vi "信息转换.vi"(7 "联机模式":enum16{"单机", "追溯"}(ring)=enum."追溯", 8 "错误输入（无错误）":errorcluster, 10 "追溯码":string[](array[string]), 11 "测试信息":T1) -> (0 "错误输出":errorcluster, 3 "信息输出":string[](array[string]))   [LabVIEW 2020]
panel:
  # "用户信息转换"
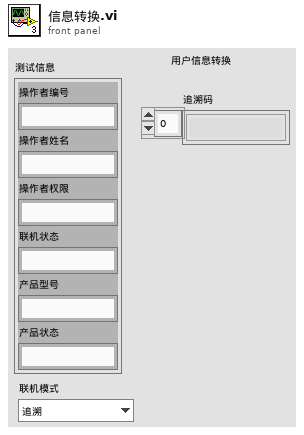
[diagram p1: front panel]
types:
  T1 = cluster{"操作者编号":string, "操作者姓名":string, "操作者权限":string, "联机状态":string, "产品型号":string, "产品状态":string}
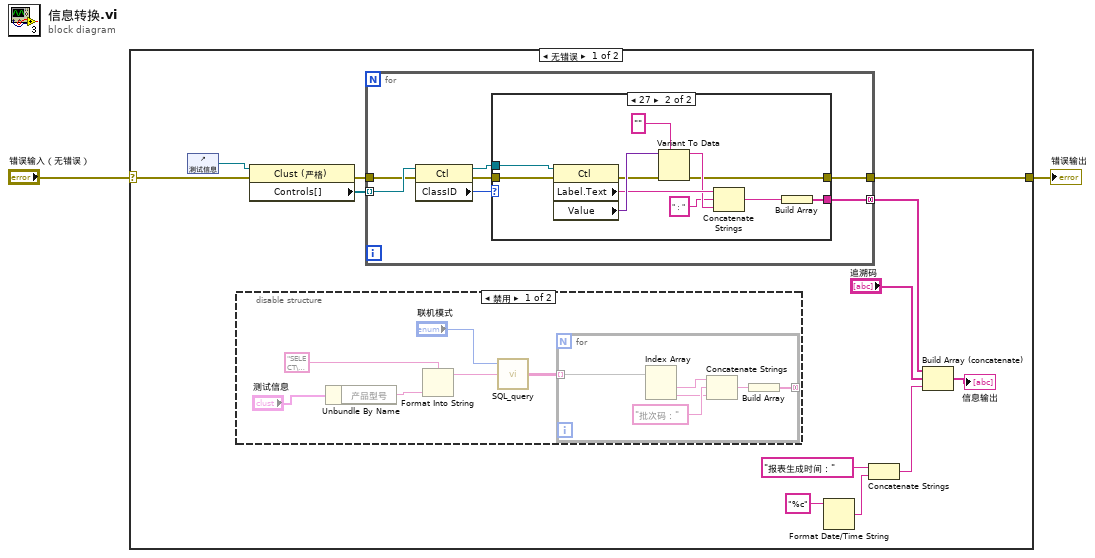
[diagram p0: block diagram]
diagram:
  n1 = case shown="无错误" "错误输入（无错误）" {
    selector: "错误输入（无错误）" -> [w7 w46]
    tunnel: [w5 w46] -> w1
    frame No Error {
      n2 = control-ref of="测试信息"() -> (w14:refnum<vi>)
      n3 = disable-structure shown="禁用" {
        frame Disabled {
          n4 = Unbundle By Name("测试信息") -> ("产品型号"=w19:string)
          n5 = Format Into String(format string="SELECT\ndbo.ProductBatch.Product,\ndbo.ProductBatch.Batch,\ndbo.ProductBatch.Remain\nFROM\ndbo.ProductBatch\nWHERE\ndbo.ProductBatch.Modle = N'%s'" ("SQL query"), w19) -> (resulting string=w18:string)  [unwired: 2 in, 1 out]
          n6 = call "SQL_query.vi"("SQL query"=w18, "联机模式"="联机模式") -> ("data"=w17:string[][])  [unwired: 2 in, 1 out]
          n7 = for {
            tunnel: w17 -> [w24] mode=indexing
            tunnel: [w21] -> _ mode=concatenating
            n8 = Index Array(array=w24) -> (element #1=w23:string, element #2=w22:string)  [unwired: 2 in]
            n9 = Concatenate Strings(w23, "批次码：" ("字符串"), w22) -> (w25:string)
            n10 = Build Array(w25) -> (w21:string[])
          }
        }
        frame Enabled {
        }
      }
      n11 = property on="属性节点" class="Clust (严格)"(reference=w14, error in=w7) -> (error out=w6:errorcluster, "Controls[]"=w13:refnum<vi>[])  [unwired: 1 out]
      n12 = for {
        tunnel: w13 -> [w33] mode=indexing
        tunnel: [w30] -> w11 mode=concatenating
        tunnel: w6 -> [w29]
        tunnel: [w27] -> w5
        n13 = property class="Ctl"(reference=w33, error in=w29) -> (reference out=w31:refnum<vi>, error out=w28:errorcluster, "ClassID"=w32:u32)
        n14 = case shown="27" w32 {
          tunnel: w31 -> [_ w45]
          tunnel: [_ w38] -> w30
          tunnel: w28 -> [w34 w37]
          tunnel: [w34 w35] -> w27
          frame 0, Default {
          }
          frame 27 {
            n15 = property class="Ctl"(reference=w45, error in=w37) -> (error out=w36:errorcluster, "Label.Text"=w42:string, "Value"=w43:variant)  [unwired: 1 out]
            n16 = Variant To Data(error in=w36, type="", Variant=w43) -> (data=w41:string, error out=w35:errorcluster)
            n17 = Concatenate Strings(w42, "：" ("字符串"), w41) -> (w39:string)
            n18 = Build Array(w39) -> (w38:string[])
          }
        }
      }
      n19 = Format Date/Time String(time format string (%c)="%c") -> (date/time string=w8:string)  [unwired: 2 in]
      n20 = Concatenate Strings("报表生成时间：" ("字符串"), w8) -> (w4:string)
      n21 = Build Array (concatenate)(w11, "追溯码", w4) -> (→"信息输出":string[])
    }
    frame Error {
    }
  }
  "错误输出" <- w1
